vi "HEWH_Elapsed Timer.vi"(8 "error in":errorcluster, 11 "Message Queues out":T2) -> (0 "error out":errorcluster)   [LabVIEW 2023]
uses:
  Tenney/support/Message Queue/All Message Queues.ctl
  Tenney/support/Message Queue/Message Cluster.ctl
  Type Definitions/HEWH Timer.ctl
  FVIR and LDO/support/Message Queue/Enqueue Message (Single).vi
  FVIR and LDO/support/Message Queue/Message Queue.lvlib
  Tenney/support/Message Queue/Tenney Message Queue.lvlib
panel:
  out "Loop Counter":i32
  out "Scan Rate (mS)":u32
  out "Timer":T1
  in  "Debug":bool
  out "Debug":string[](array[string])
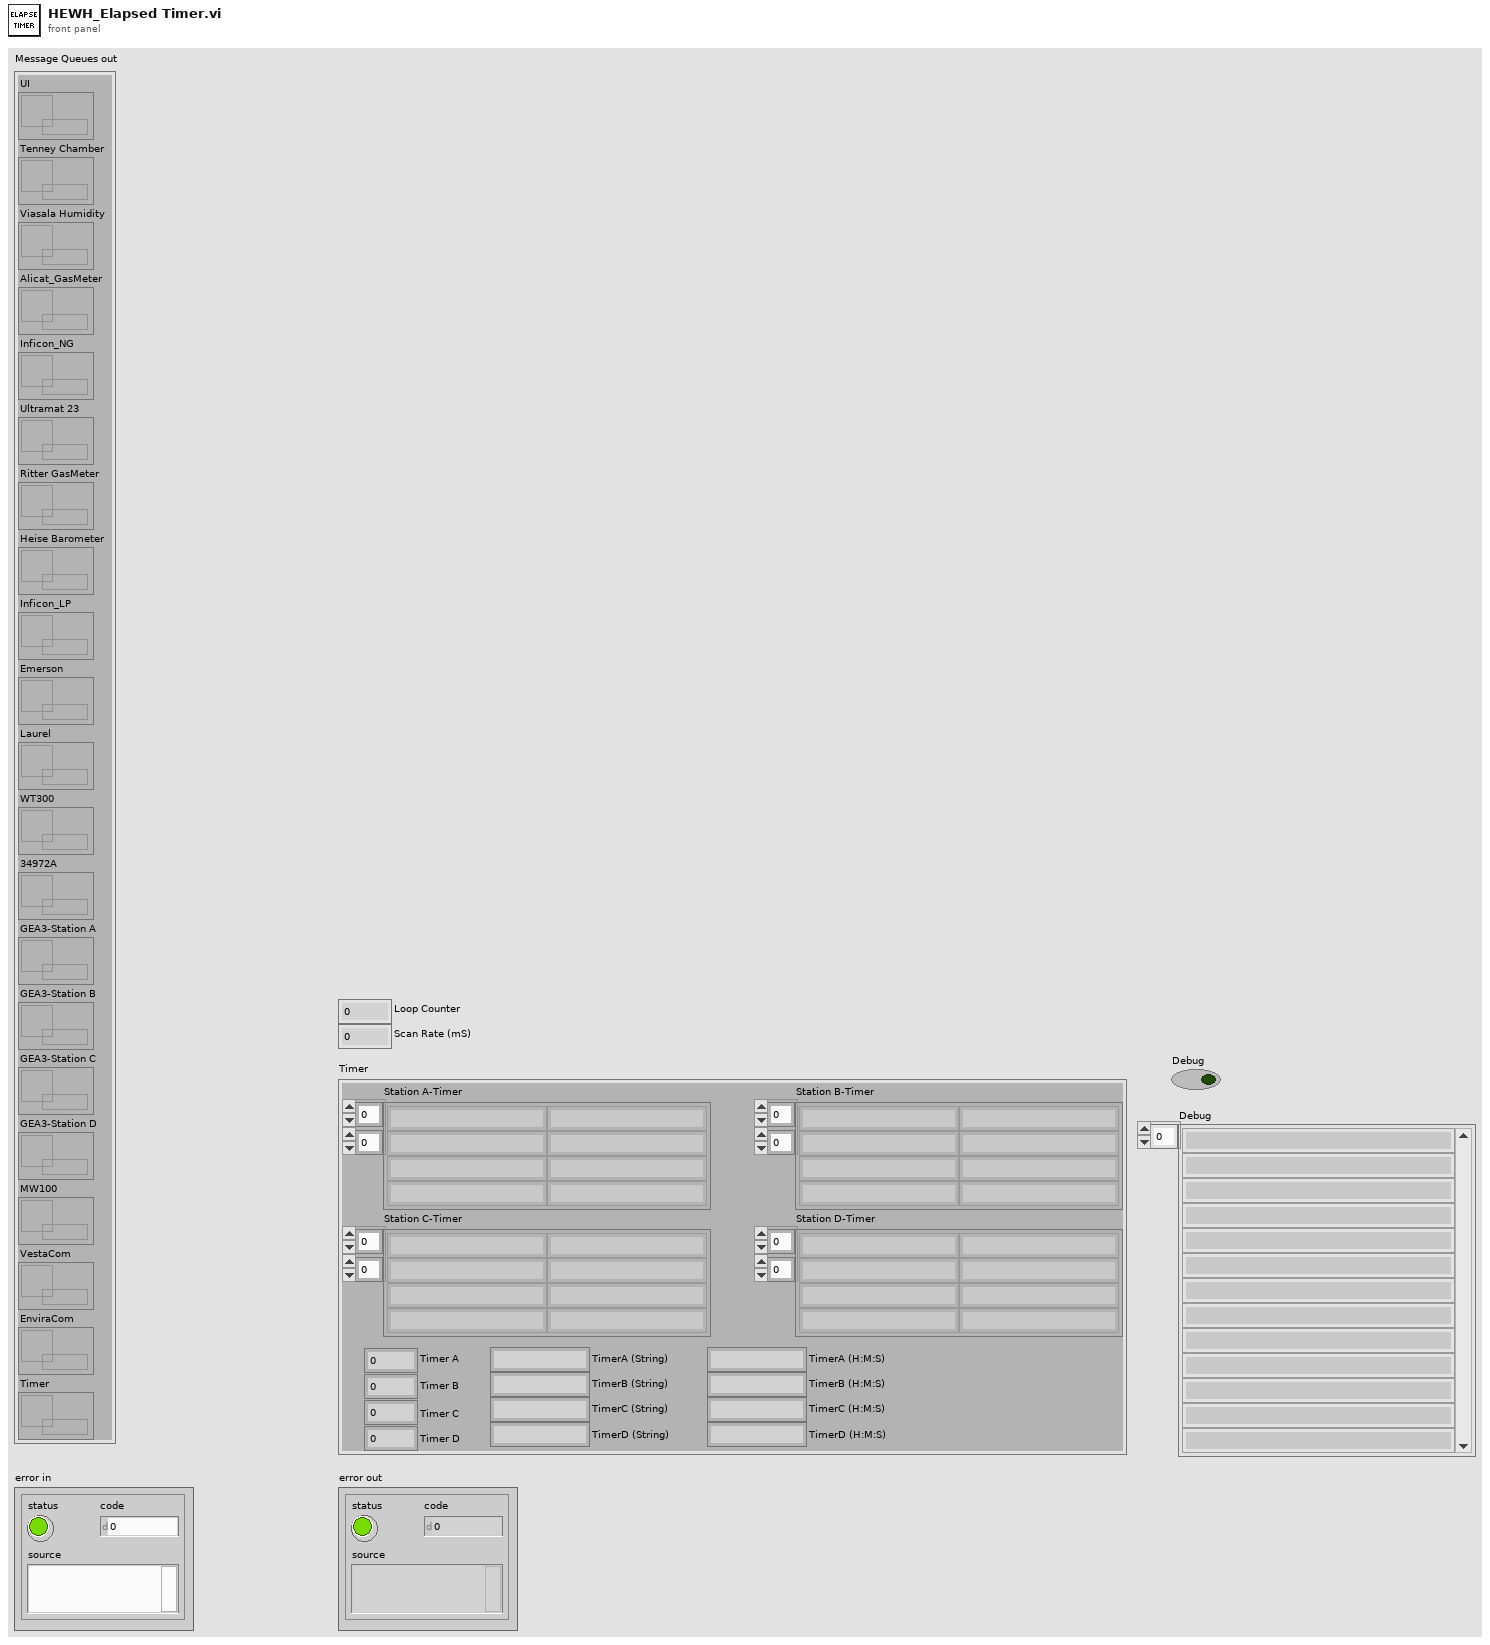
[diagram p1: front panel]
types:
  T1 = typedef "HEWH Timer.ctl" = cluster{"Station A-Timer":string[][], "Station B-Timer":string[][], "Station C-Timer":string[][], "Station D-Timer":string[][], "Timer A":dbl, "Timer B":dbl, "Timer C":dbl, "Timer D":dbl, "TimerA (String)":string, "TimerB (String)":string, "TimerC (String)":string, "TimerD (String)":string, "TimerA (H:M:S)":string, "TimerB (H:M:S)":string, "TimerC (H:M:S)":string, "TimerD (H:M:S)":string}
  T2 = typedef "Tenney Message Queue.lvlib/All Message Queues.ctl" = cluster{"UI":refnum<queue>, "Tenney Chamber":refnum<queue>, "Viasala Humidity":refnum<queue>, "Alicat_GasMeter":refnum<queue>, "Inficon_NG":refnum<queue>, "Ultramat 23":refnum<queue>, "Ritter GasMeter":refnum<queue>, "Heise Barometer":refnum<queue>, "Inficon_LP":refnum<queue>, "Emerson":refnum<queue>, "Laurel":refnum<queue>, "WT300":refnum<queue>, "34972A":refnum<queue>, "GEA3-Station A":refnum<queue>, "GEA3-Station B":refnum<queue>, "GEA3-Station C":refnum<queue>, "GEA3-Station D":refnum<queue>, "MW100":refnum<queue>, "VestaCom":refnum<queue>, "EnviraCom":refnum<queue>, "Timer":refnum<queue>}
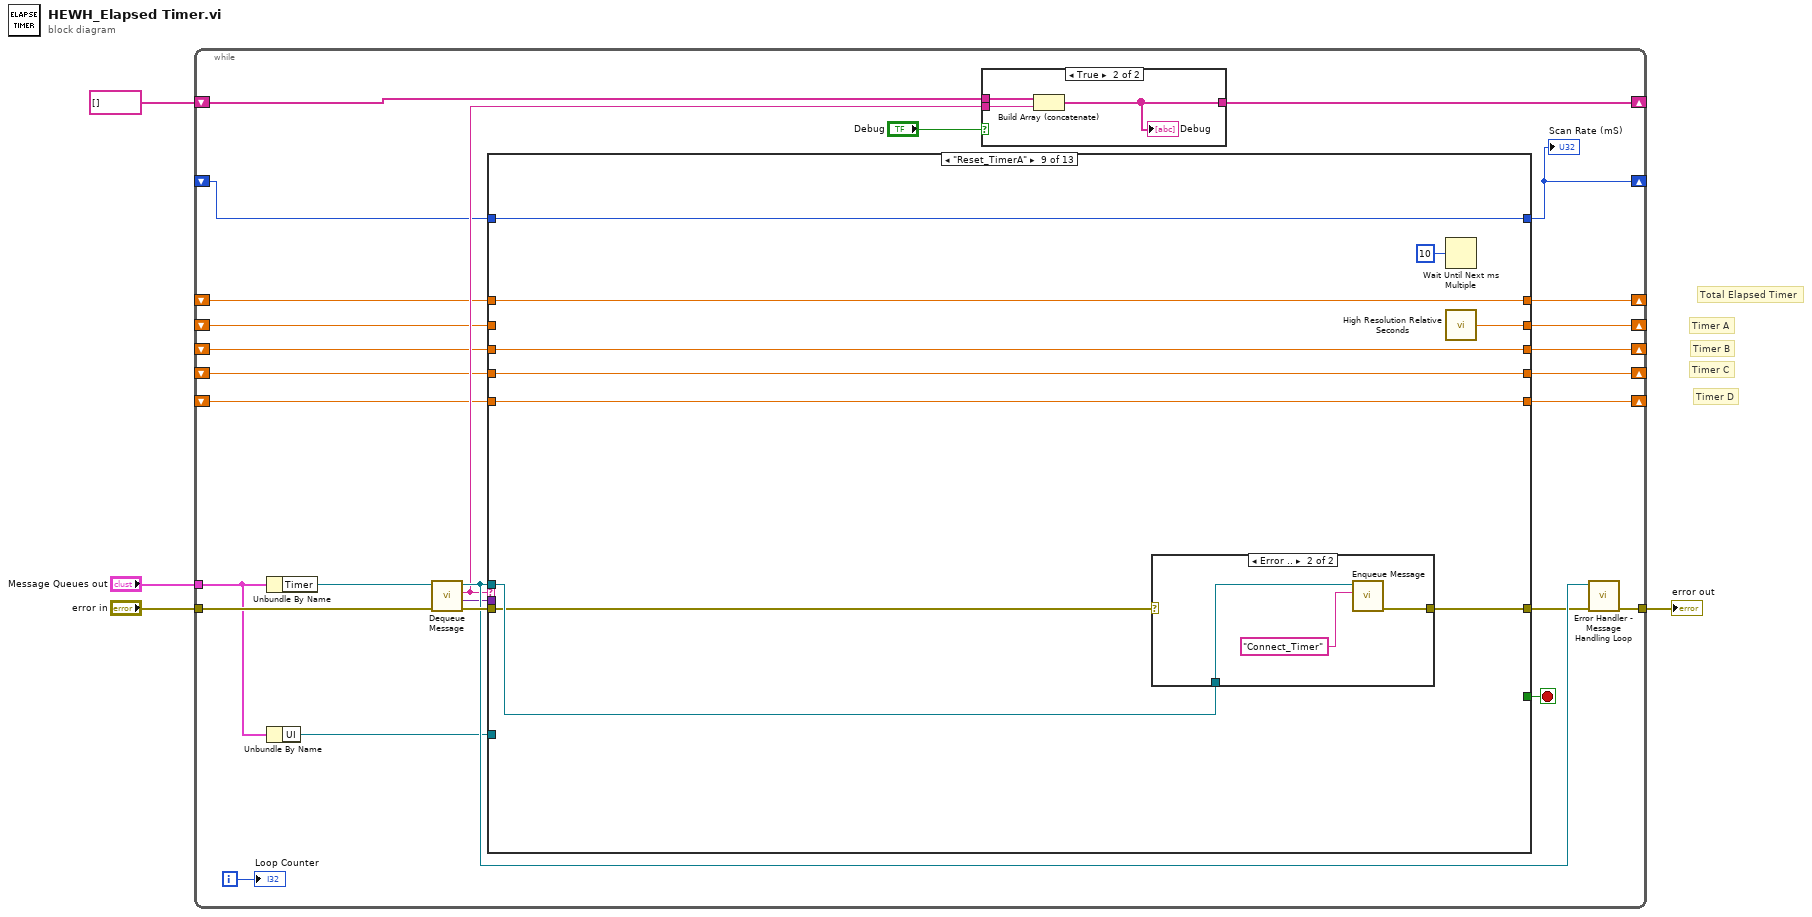
[diagram p0: block diagram]
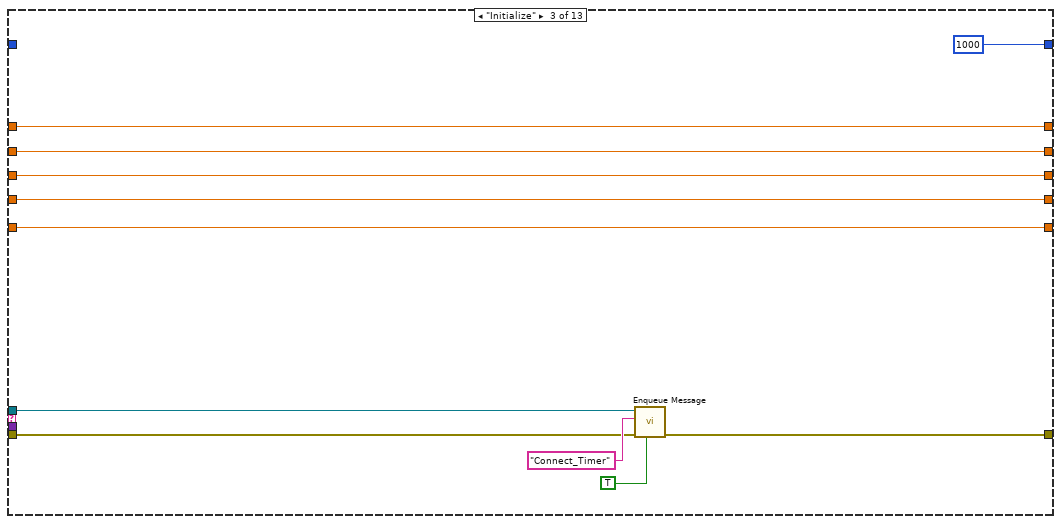
[diagram p5: hidden frame]
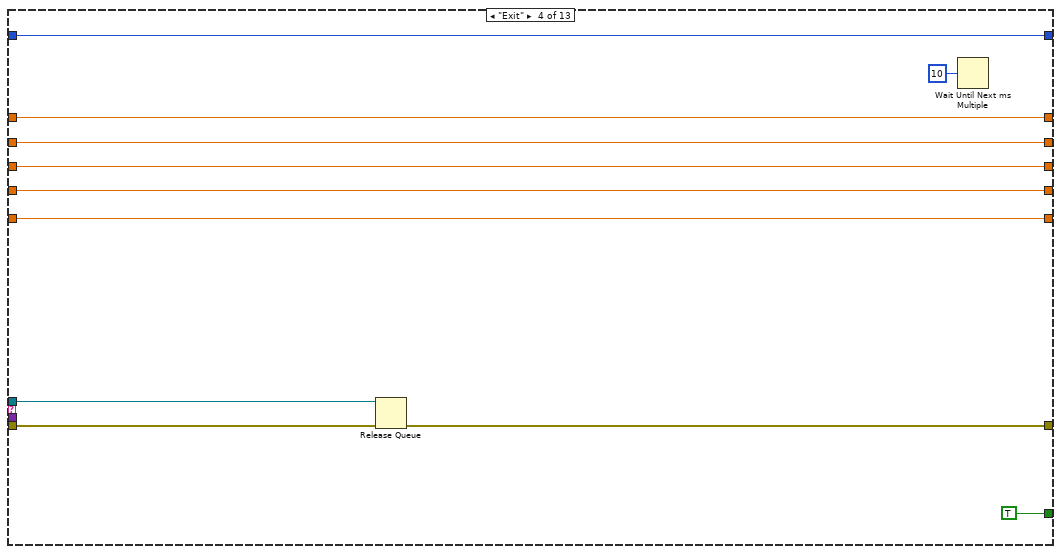
[diagram p6: hidden frame]
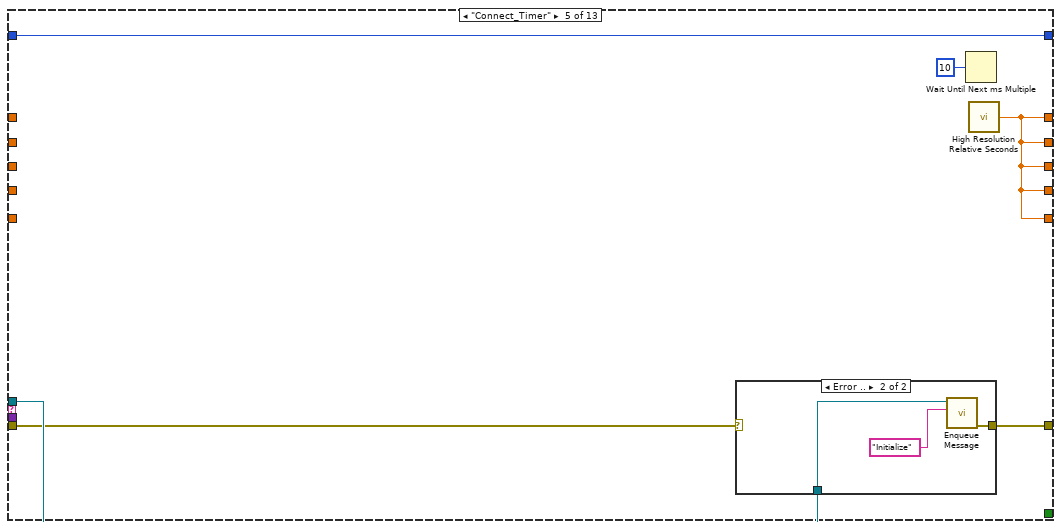
[diagram p7: hidden frame]
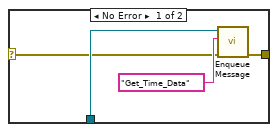
[diagram p8: hidden frame]
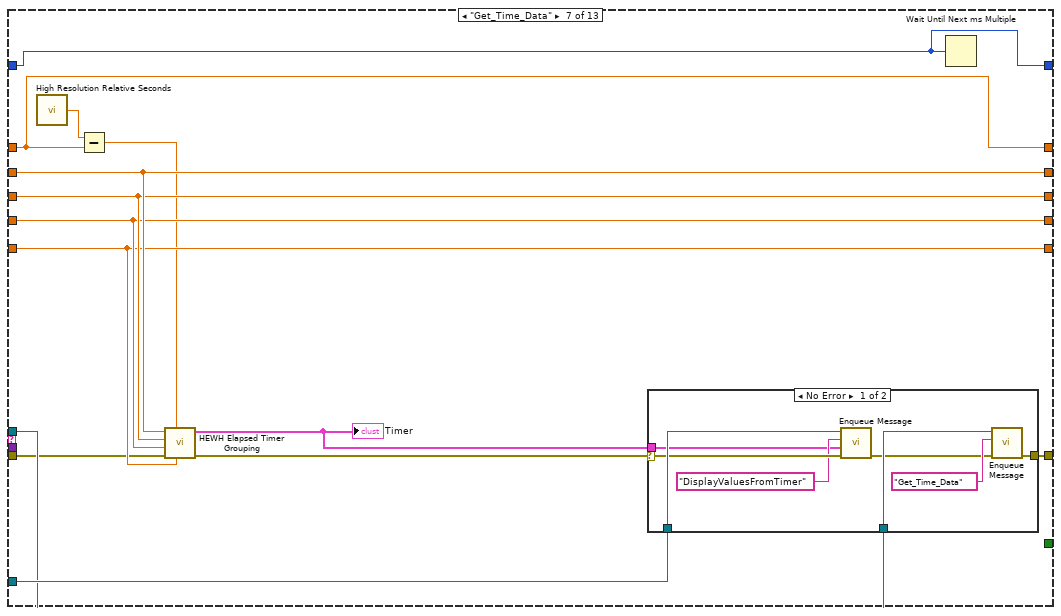
[diagram p10: hidden frame]
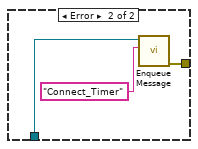
[diagram p11: hidden frame]
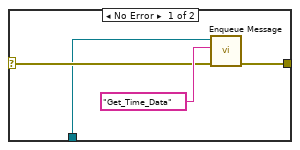
[diagram p13: hidden frame]
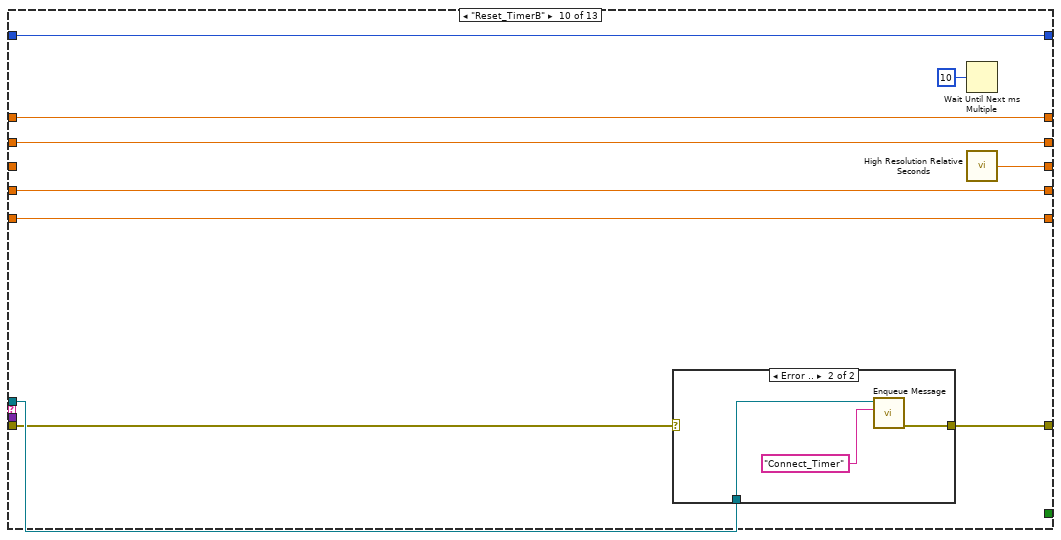
[diagram p14: hidden frame]
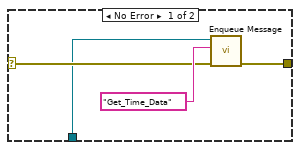
[diagram p15: hidden frame]
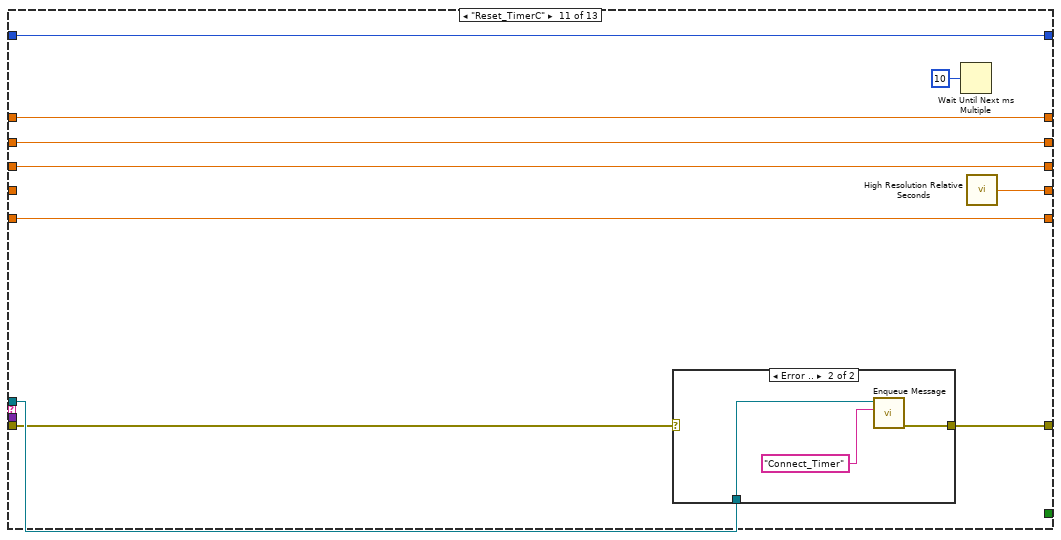
[diagram p16: hidden frame]
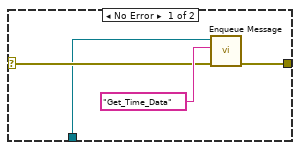
[diagram p17: hidden frame]
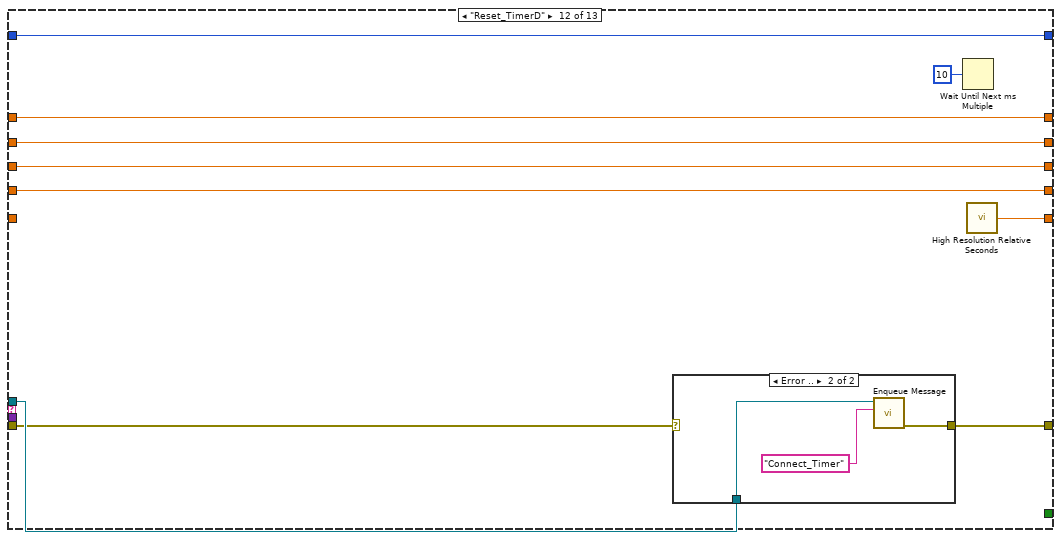
[diagram p18: hidden frame]
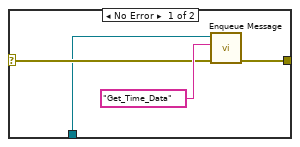
[diagram p19: hidden frame]
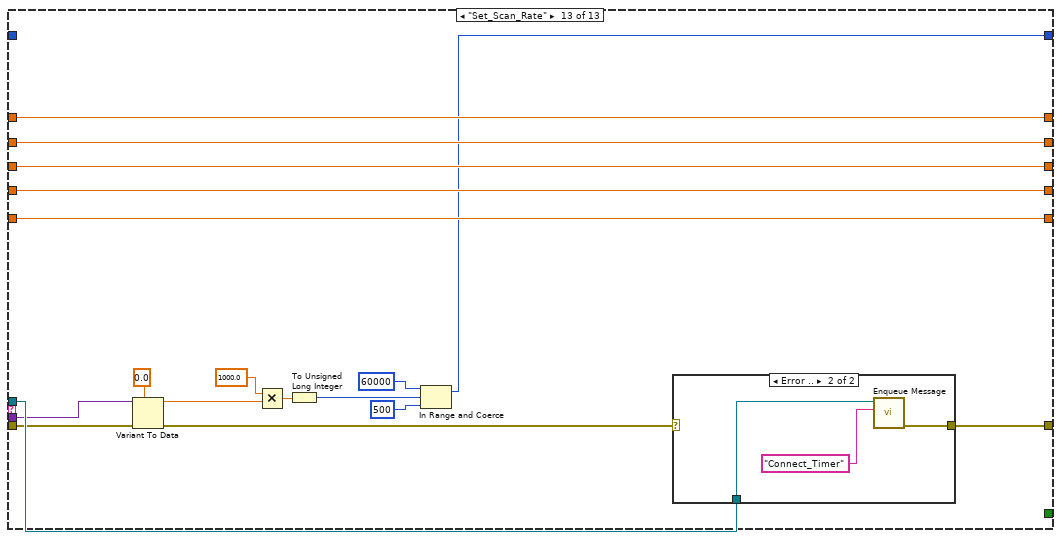
[diagram p20: hidden frame]
diagram:
  # "Total Elapsed Timer"
  # "Timer D"
  # "Timer C"
  # "Timer B"
  # "Timer A"
  n1 = while {
    tunnel: "Message Queues out" -> [w24]
    tunnel: "error in" -> [w30]
    tunnel: [w26] -> w3
    shift-right: [w20] -> _
    shift-left: string[] [] -> [w21]
    shift-right: [w17] -> _
    shift-left: _ -> [w16]
    shift-right: [w15] -> _
    shift-left: _ -> [w12]
    shift-right: [w14] -> _
    shift-left: _ -> [w11]
    shift-right: [w13] -> _
    shift-left: _ -> [w10]
    shift-right: [w9] -> _
    shift-left: _ -> [w8]
    shift-right: [w5] -> _
    shift-left: _ -> [w7]
    i -> [w6]
    stop <- w28 stop-if-true
    n2 = Unbundle By Name(w24) -> ("Timer"=w31:refnum<queue>)
    n3 = Unbundle By Name(w24) -> ("UI"=w23:refnum<queue>)
    n4 = call "Dequeue Message.vi"("error in (no error)"=w30, "Message Queue"=w31) -> ("error out"=w29:errorcluster, "Message Data"=w18:variant, "Message"=w22:string, "dup Message Queue"=w27:refnum<queue>)  [unwired: 6 in]
    n5 = case shown="\"Reset_TimerA\"" w22 {
      tunnel: w29 -> [w37 w44 w59 w69 w75 w86 w96 w118 w126 w148 w165 w182 w202]
      tunnel: [w37 w44 w58 w68 w77 w86 w104 w118 w133 w150 w167 w184 w209] -> w25
      tunnel: [_ _ _ TRUE _ _ _ _ _ _ _ _ _] -> w28
      tunnel: w27 -> [_ _ w57 w70 w76 _ w103 _ w132 w149 w166 w183 w208]
      tunnel: w23 -> [_ _ _ _ _ _ w105 _ _ _ _ _ _]
      tunnel: w18 -> [_ _ _ _ _ _ _ _ _ _ _ _ w199]
      tunnel: [w41 w48 w54 w66 w74 w90 w102 w122 w131 w146 w163 w180 w207] -> w17
      tunnel: w16 -> [w41 w48 w54 w66 _ w90 w102 w122 _ w146 w163 w180 w207]
      tunnel: [w40 w47 w53 w65 w74 w89 w101 w121 w130 w147 w162 w179 w206] -> w15
      tunnel: [w39 w46 w52 w64 w74 w88 w100 w120 w129 w145 w164 w178 w205] -> w14
      tunnel: [w38 w45 w51 w63 w74 w87 w99 w119 w128 w144 w161 w181 w203] -> w13
      tunnel: w12 -> [w40 w47 w53 w65 _ w89 w101 w121 w130 _ w162 w179 w206]
      tunnel: w11 -> [w39 w46 w52 w64 _ w88 w100 w120 w129 w145 _ w178 w205]
      tunnel: w10 -> [w38 w45 w51 w63 _ w87 w99 w119 w128 w144 w161 _ w203]
      tunnel: [w42 w49 w55 w67 w74 w91 w97 w123 w127 w143 w160 w177 w204] -> w9
      tunnel: w8 -> [w42 w49 w55 w67 _ w91 w97 w123 w127 w143 w160 w177 w204]
      tunnel: [w36 w43 u32 1000 ("millisecond multiple") w62 w73 w85 w92 w117 w125 w142 w159 w176 w192] -> w5
      tunnel: w7 -> [w36 w43 _ w62 w73 w85 w92 w117 w125 w142 w159 w176 _]
      frame "---------- Setup ----------" {
      }
      frame Default {
      }
      frame "Initialize" {
        n6 = call-poly "Enqueue Message.vi"("Priority Message? (F)"=TRUE, "error in (no error)"=w59, "Message"="Connect_Timer", "Message Queue"=w57) -> ("error out"=w58:errorcluster)  [unwired: 6 in, 1 out]
      }
      frame "Exit" {
        n7 = Release Queue(queue=w70, error in (no error)=w69) -> (error out=w68:errorcluster)  [unwired: 1 in, 2 out]
        n8 = Wait Until Next ms Multiple(millisecond multiple=u32 10) -> ()  [unwired: 1 out]
      }
      frame "Connect_Timer" {
        n9 = case shown="Error .." w75 {
          selector: w75 -> [w78 _]
          tunnel: [w80 w83] -> w77
          tunnel: w76 -> [w79 w82]
          frame No Error {
            n10 = call-poly "Enqueue Message.vi"("error in (no error)"=w78, "Message"="Get_Time_Data", "Message Queue"=w79) -> ("error out"=w80:errorcluster)  [unwired: 7 in, 1 out]
          }
          frame Error {
            n11 = call-poly "Enqueue Message.vi"("Message"="Initialize", "Message Queue"=w82) -> ("error out"=w83:errorcluster)  [unwired: 8 in, 1 out]
          }
        }
        n12 = Wait Until Next ms Multiple(millisecond multiple=u32 10) -> ()  [unwired: 1 out]
        n13 = call <vilib>:"High Resolution Relative Seconds.vi"() -> ("relative seconds"=w74:dbl)
      }
      frame "---------- Data Collection ----------" {
      }
      frame "Get_Time_Data" {
        n14 = call <vilib>:"High Resolution Relative Seconds.vi"() -> ("relative seconds"=w98:dbl)
        n15 = Subtract(x=w98, y=w97) -> (x-y=w94:dbl)
        n16 = call "HEWH Elapsed Timer Grouping.vi"("Timer D"=w99, "Total Elapsed Time"=w94, "error in (no error)"=w96, "Timer C"=w100, "Timer B"=w101, "Timer A"=w102) -> ("error out"=w95:errorcluster, "Timer"=w93:T1)  [unwired: 4 in]
        "Timer" <- w93
        n17 = case shown="No Error" w95 {
          selector: w95 -> [w108 _]
          tunnel: w105 -> [w113 _]
          tunnel: [w112 w115] -> w104
          tunnel: w103 -> [w111 w114]
          tunnel: w93 -> [w106 _]
          frame No Error {
            n18 = call-poly "Enqueue Message.vi"("error in (no error)"=w108, "Message Data"=w106, "Message"="DisplayValuesFromTimer", "Message Queue"=w113) -> ("error out"=w109:errorcluster)  [unwired: 6 in, 1 out]
            n19 = call-poly "Enqueue Message.vi"("error in (no error)"=w109, "Message"="Get_Time_Data", "Message Queue"=w111) -> ("error out"=w112:errorcluster)  [unwired: 7 in, 1 out]
          }
          frame Error {
            n20 = call-poly "Enqueue Message.vi"("Message"="Connect_Timer", "Message Queue"=w114) -> ("error out"=w115:errorcluster)  [unwired: 8 in, 1 out]
          }
        }
        n21 = Wait Until Next ms Multiple(millisecond multiple=w92) -> ()  [unwired: 1 out]
      }
      frame "---------- Timer Control ----------" {
      }
      frame "Reset_TimerA" {
        n22 = case shown="Error .." w126 {
          selector: w126 -> [w136 _]
          tunnel: [w135 w139] -> w133
          tunnel: w132 -> [w134 w138]
          frame No Error {
            n23 = call-poly "Enqueue Message.vi"("error in (no error)"=w136, "Message"="Get_Time_Data", "Message Queue"=w134) -> ("error out"=w135:errorcluster)  [unwired: 7 in, 1 out]
          }
          frame Error {
            n24 = call-poly "Enqueue Message.vi"("Message"="Connect_Timer", "Message Queue"=w138) -> ("error out"=w139:errorcluster)  [unwired: 8 in, 1 out]
          }
        }
        n25 = Wait Until Next ms Multiple(millisecond multiple=u32 10) -> ()  [unwired: 1 out]
        n26 = call <vilib>:"High Resolution Relative Seconds.vi"() -> ("relative seconds"=w131:dbl)
      }
      frame "Reset_TimerB" {
        n27 = case shown="Error .." w148 {
          selector: w148 -> [w153 _]
          tunnel: [w152 w156] -> w150
          tunnel: w149 -> [w151 w155]
          frame No Error {
            n28 = call-poly "Enqueue Message.vi"("error in (no error)"=w153, "Message"="Get_Time_Data", "Message Queue"=w151) -> ("error out"=w152:errorcluster)  [unwired: 7 in, 1 out]
          }
          frame Error {
            n29 = call-poly "Enqueue Message.vi"("Message"="Connect_Timer", "Message Queue"=w155) -> ("error out"=w156:errorcluster)  [unwired: 8 in, 1 out]
          }
        }
        n30 = Wait Until Next ms Multiple(millisecond multiple=u32 10) -> ()  [unwired: 1 out]
        n31 = call <vilib>:"High Resolution Relative Seconds.vi"() -> ("relative seconds"=w147:dbl)
      }
      frame "Reset_TimerC" {
        n32 = case shown="Error .." w165 {
          selector: w165 -> [w170 _]
          tunnel: [w169 w173] -> w167
          tunnel: w166 -> [w168 w172]
          frame No Error {
            n33 = call-poly "Enqueue Message.vi"("error in (no error)"=w170, "Message"="Get_Time_Data", "Message Queue"=w168) -> ("error out"=w169:errorcluster)  [unwired: 7 in, 1 out]
          }
          frame Error {
            n34 = call-poly "Enqueue Message.vi"("Message"="Connect_Timer", "Message Queue"=w172) -> ("error out"=w173:errorcluster)  [unwired: 8 in, 1 out]
          }
        }
        n35 = Wait Until Next ms Multiple(millisecond multiple=u32 10) -> ()  [unwired: 1 out]
        n36 = call <vilib>:"High Resolution Relative Seconds.vi"() -> ("relative seconds"=w164:dbl)
      }
      frame "Reset_TimerD" {
        n37 = case shown="Error .." w182 {
          selector: w182 -> [w187 _]
          tunnel: [w186 w190] -> w184
          tunnel: w183 -> [w185 w189]
          frame No Error {
            n38 = call-poly "Enqueue Message.vi"("error in (no error)"=w187, "Message"="Get_Time_Data", "Message Queue"=w185) -> ("error out"=w186:errorcluster)  [unwired: 7 in, 1 out]
          }
          frame Error {
            n39 = call-poly "Enqueue Message.vi"("Message"="Connect_Timer", "Message Queue"=w189) -> ("error out"=w190:errorcluster)  [unwired: 8 in, 1 out]
          }
        }
        n40 = Wait Until Next ms Multiple(millisecond multiple=u32 10) -> ()  [unwired: 1 out]
        n41 = call <vilib>:"High Resolution Relative Seconds.vi"() -> ("relative seconds"=w181:dbl)
      }
      frame "Set_Scan_Rate" {
        n42 = Variant To Data(error in=w202, type=0.0 ("millisecond multiple"), Variant=w199) -> (data=w193:dbl, error out=w201:errorcluster)
        n43 = Multiply(x=1000.0 ("y"), y=w193) -> (x*y=w197:dbl)
        n44 = To Unsigned Long Integer(number=w197) -> (unsigned 32bit integer=w198:u32)
        n45 = In Range and Coerce(upper limit=u32 60000, x=w198, lower limit=u32 500) -> (coerced(x)=w192:u32)  [unwired: 1 out]
        n46 = case shown="Error .." w201 {
          selector: w201 -> [w212 _]
          tunnel: [w211 w215] -> w209
          tunnel: w208 -> [w210 w214]
          frame No Error {
            n47 = call-poly "Enqueue Message.vi"("error in (no error)"=w212, "Message"="Get_Time_Data", "Message Queue"=w210) -> ("error out"=w211:errorcluster)  [unwired: 7 in, 1 out]
          }
          frame Error {
            n48 = call-poly "Enqueue Message.vi"("Message"="Connect_Timer", "Message Queue"=w214) -> ("error out"=w215:errorcluster)  [unwired: 8 in, 1 out]
          }
        }
      }
    }
    "Scan Rate (mS)" <- w5
    n49 = case shown="True" "Debug" {
      tunnel: w22 -> [_ w35]
      tunnel: w21 -> [w32 w34]
      tunnel: [w32 w33] -> w20
      frame False {
      }
      frame True {
        n50 = Build Array (concatenate)(w34, w35) -> (w33:string[])
        "Debug" <- w33
      }
    }
    n51 = call "Error Handler - Message Handling Loop.vi"("error in (no error)"=w25, "Message Queue"=w27) -> ("dup error in"=w26:errorcluster)  [unwired: 8 in, 1 out]
    "Loop Counter" <- w6
  }
  "error out" <- w3
